vi "CIE-Plot Data.vi"(0 "Path":path, 5 "Mag graph":refnum<vi>, 7 "Phase graph":refnum<vi>, 9 "Tolerance (dB)":dbl=10.0, 11 "error in":errorcluster, 12 "Plot Max SPL (F)":bool) -> (4 "Path (out)":path, 15 "error out":errorcluster)   [LabVIEW 2015]
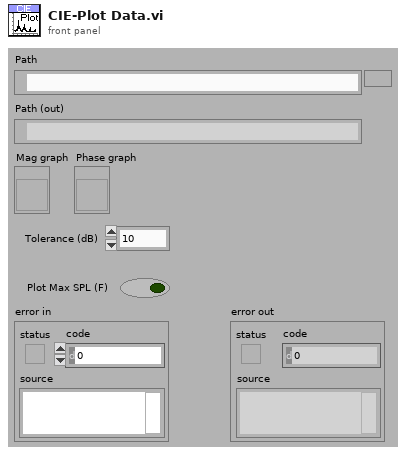
[diagram p1: front panel]
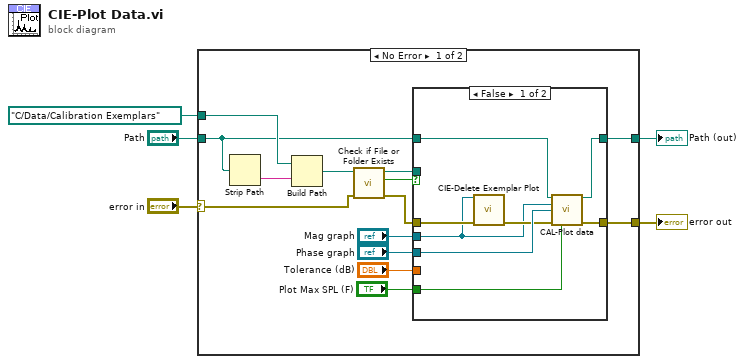
[diagram p0: block diagram]
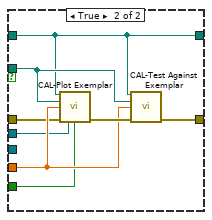
[diagram p2: hidden frame]
diagram:
  n1 = case shown="No Error" "error in" {
    selector: "error in" -> [w7 w37]
    tunnel: path "C:/Data/Calibration Exemplars" ("base path") -> [w18 _]
    tunnel: "Path" -> [w14 w36]
    tunnel: [w10 w36] -> w3
    tunnel: [w8 w37] -> w2
    frame No Error {
      n2 = Strip Path(path=w14) -> (name=w19:string)  [unwired: 1 out]
      n3 = Build Path(base path=w18, name or relative path=w19) -> (appended path=w17:path)
      n4 = call <vilib>:"Check if File or Folder Exists.vi"("error in (no error)"=w7, "path"=w17) -> ("error out"=w9:errorcluster, "file or folder exists?"=w16:bool, "dup path"=w15:path)  [unwired: 7 in]
      n5 = case shown="False" w16 {
        tunnel: w15 -> [_ w34]
        tunnel: w14 -> [w27 w31]
        tunnel: "Tolerance (dB)" -> [_ w33]
        tunnel: "Mag graph" -> [w20 w32]
        tunnel: "Phase graph" -> [w26 _]
        tunnel: [w25 w31] -> w10
        tunnel: w9 -> [w22 w30]
        tunnel: [w24 w29] -> w8
        tunnel: "Plot Max SPL (F)" -> [w23 w28]
        frame False {
          n6 = call "CIE-Delete Exemplar Plot.vi"("Mag graph"=w20, "error in (no error)"=w22) -> ("error out"=w21:errorcluster)  [unwired: 13 in]
          n7 = call "CAL-Plot data.vi"("Path"=w27, "Mag graph"=w20, "Phase graph"=w26, "error in (no error)"=w21, "Plot Max SPL (F)"=w23) -> ("Path (out)"=w25:path, "error out"=w24:errorcluster)  [unwired: 9 in]
        }
        frame True {
          n8 = call "CAL-Plot Exemplar.vi"("Test file"=w31, "Exemplar file"=w34, "Tolerance (dB)"=w33, "error in"=w30, "Magnitude graph ref"=w32, "Max SPL?"=w28) -> ("error out"=w35:errorcluster)  [unwired: 9 in]
          n9 = call "CAL-Test Against Exemplar.vi"("Test file"=w31, "Exemplar file"=w34, "Tolerance (dB)"=w33, "error in"=w35) -> ("error out"=w29:errorcluster)  [unwired: 11 in]
        }
      }
    }
    frame Error {
    }
  }
  "error out" <- w2
  "Path (out)" <- w3
